vi "Post-Install Custom Action.vi"(10 "Variant":variant) -> (0 "error out":errorcluster)   [LabVIEW 2016]
uses:
  <vilib>/Utility/traverseref.llb/TRef TravTarget.ctl
  <vilib>/Utility/traverseref.llb/VI Scripting - Traverse.lvlib
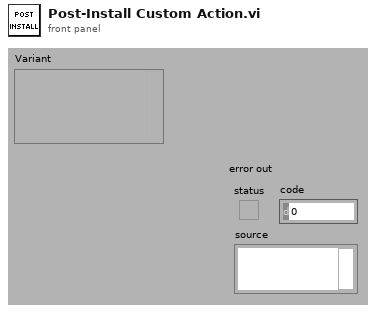
[diagram p1: front panel]
types:
  T1 = enum32{"Invalid", "Standard", "Closed", "Hidden", "Minimized", "Maximized"}
  T2 = typedef "TRef TravTarget.ctl" = enum16{"FP", "BD", "Other"}
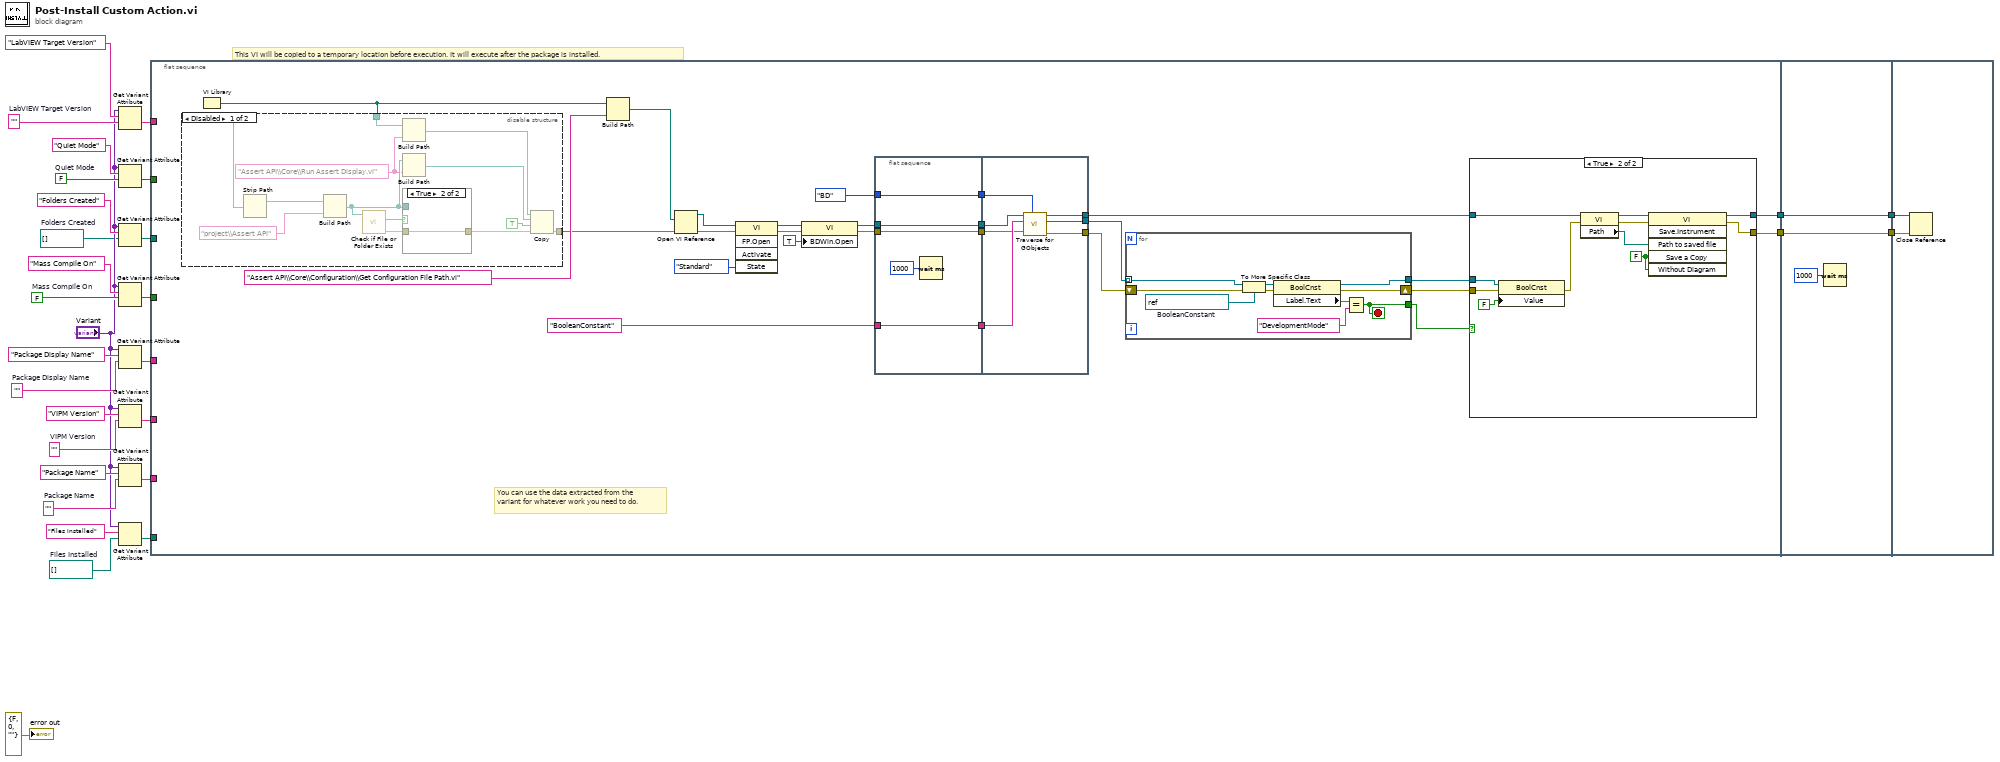
[diagram p0: block diagram]
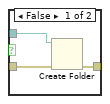
[diagram p2: hidden frame]
diagram:
  w5 = path[] []  # Folders Created
  w6 = path[] []  # Files Installed
  w12 = FALSE  # Mass Compile On
  w13 = ""  # Package Display Name
  w20 = FALSE  # Quiet Mode
  w23 = ""  # VIPM Version
  w25 = ""  # LabVIEW Target Version
  w27 = ""  # Package Name
  # "This VI will be copied to a temporary location before execution. It will execute after the package is installed."
  n1 = Get Variant Attribute(Variant="Variant", name="LabVIEW Target Version", default value (empty Variant)=w25) -> (value=w17:string)  [unwired: 1 in, 3 out]
  n2 = Get Variant Attribute(Variant="Variant", name="Quiet Mode", default value (empty Variant)=w20) -> (value=w15:bool)  [unwired: 1 in, 3 out]
  n3 = Get Variant Attribute(Variant="Variant", name="Folders Created", default value (empty Variant)=w5) -> (value=w10:path[])  [unwired: 1 in, 3 out]
  n4 = Get Variant Attribute(Variant="Variant", name="Mass Compile On", default value (empty Variant)=w12) -> (value=w14:bool)  [unwired: 1 in, 3 out]
  n5 = Get Variant Attribute(Variant="Variant", name="Package Display Name", default value (empty Variant)=w13) -> (value=w19:string)  [unwired: 1 in, 3 out]
  n6 = Get Variant Attribute(Variant="Variant", name="VIPM Version", default value (empty Variant)=w23) -> (value=w16:string)  [unwired: 1 in, 3 out]
  n7 = Get Variant Attribute(Variant="Variant", name="Package Name", default value (empty Variant)=w27) -> (value=w18:string)  [unwired: 1 in, 3 out]
  n8 = Get Variant Attribute(Variant="Variant", name="Files Installed", default value (empty Variant)=w6) -> (value=w9:path[])  [unwired: 1 in, 3 out]
  n9 = flat-sequence {
    tunnel: w19 -> [_]
    tunnel: w18 -> [_]
    tunnel: w17 -> [_]
    tunnel: w16 -> [_]
    tunnel: w15 -> [_]
    tunnel: w14 -> [_]
    tunnel: w9 -> [_]
    tunnel: w10 -> [_]
    tunnel: [w40] -> w3
    tunnel: [w39] -> w2
    tunnel: [w110] -> w4
    tunnel: w3 -> [w110]
    tunnel: w2 -> [w109]
    tunnel: [w109] -> w1
    tunnel: w4 -> [w112]
    tunnel: w1 -> [w111]
    frame #0 {
      # "Quiet Mode: This will indicate if VIPM is working in quiet mode.\nThis may happen if VIPM is running silently from the VIPM API.\nIf this is true then you should respect quiet mode and perform\nactions without any blocking dialog boxes or user prompts."
      # "You can use the data extracted from the variant for whatever work you need to do."
      n10 = VI Library() -> (path=w56:path)
      n11 = disable-structure shown="Disabled" {
        disable-tunnel: w56 -> [w70 _]
        disable-tunnel: [w69 _] -> w53
        frame Disabled {
          w75 = "Assert API\\Core\\Run Assert Display.vi" ("name or relative path")
          n12 = Strip Path(path=w70) -> (stripped path=w71:path)  [unwired: 1 out]
          n13 = Build Path(base path=w71, name or relative path="project\\Assert API") -> (appended path=w76:path)
          n14 = call <vilib>:"Check if File or Folder Exists.vi"("path"=w76) -> ("error out"=w77:errorcluster, "file or folder exists?"=w78:bool)  [unwired: 8 in, 1 out]
          n15 = Build Path(base path=w70, name or relative path=w75) -> (appended path=w80:path)
          n16 = Build Path(base path=w76, name or relative path=w75) -> (appended path=w74:path)
          n17 = case shown="True" w78 {
            tunnel: w76 -> [w83 _]
            tunnel: w77 -> [w82 w84]
            tunnel: [w81 w84] -> w72
            frame False {
              n18 = Create Folder(path (use dialog)=w83, error in=w82) -> (error out=w81:errorcluster)  [unwired: 1 in, 2 out]
            }
            frame True {
            }
          }
          n19 = Copy(8:w72, 9:TRUE ("overwrite (F)"), 10:w74, 11:w80) -> (0:w69:errorcluster)  [unwired: 1 in, 2 out]
        }
        frame Enabled {
        }
      }
      n20 = Build Path(base path=w56, name or relative path="Assert API\\Core\\Configuration\\Get Configuration File Path.vi") -> (appended path=w54:path)
      n21 = Open VI Reference(vi path=w54, error in (no error)=w53) -> (vi reference=w42:refnum<vi>, error out=w52:errorcluster)  [unwired: 4 in]
      n22 = invoke class="VI" method="FP.Open"(reference=w42, error in=w52, "State"=T1."Standard") -> (reference out=w37:refnum<vi>, error out=w43:errorcluster)  [unwired: 2 in, 3 out]
      n23 = property class="VI"(reference=w37, error in=w43, "BDWin.Open"=TRUE ("Block Diagram Window:Open")) -> (reference out=w36:refnum<vi>, error out=w38:errorcluster)
      n24 = flat-sequence {
        tunnel: w36 -> [w58]
        tunnel: w38 -> [w59]
        tunnel: "BooleanConstant" ("Class Name") -> [w60]
        tunnel: TRef_TravTarget."BD" ("Traverse Target") -> [w61]
        tunnel: [w61] -> w34
        tunnel: [w60] -> w33
        tunnel: [w59] -> w32
        tunnel: [w58] -> w31
        tunnel: [w66] -> w49
        tunnel: [w65] -> w45
        tunnel: [w64] -> w44
        tunnel: w34 -> [w68]
        tunnel: w33 -> [w67]
        tunnel: w32 -> [w63]
        tunnel: w31 -> [w62]
        frame #0 {
          n25 = Wait (ms)(milliseconds to wait=u32 1000) -> ()  [unwired: 1 out]
        }
        frame #1 {
          n26 = call <vilib>:"Traverse for GObjects.vi"("Traverse Target"=w68, "error in (no error)"=w63, "Class Name"=w67, "VI Refnum"=w62) -> ("error out"=w65:errorcluster, "References"=w66:refnum<vi>[], "dup VI Refnum"=w64:refnum<vi>)  [unwired: 4 in, 1 out]
        }
      }
      n27 = for {
        tunnel: w49 -> [w107] mode=indexing
        tunnel: [w102] -> w47
        tunnel: [w101] -> w48
        shift-right: [w100] -> w46
        shift-left: w45 -> [w99]
        stop <- w101 stop-if-true
        w105 = refnum<vi> refnum  # BooleanConstant
        n28 = To More Specific Class(target class=w105, reference=w107, error in=w99) -> (specific class reference=w106:refnum<vi>, error out=w98:errorcluster)
        n29 = property class="BoolCnst"(reference=w106, error in=w98) -> (reference out=w102:refnum<vi>, error out=w100:errorcluster, "Label.Text"=w104:string)
        n30 = Equal?(x=w104, y="DevelopmentMode") -> (x = y?=w101:bool)
      }
      n31 = case shown="True" w48 {
        tunnel: w47 -> [_ w97]
        tunnel: w46 -> [w85 w95]
        tunnel: w44 -> [w86 w94]
        tunnel: [w85 w88] -> w39
        tunnel: [w86 w87] -> w40
        frame False {
        }
        frame True {
          w89 = FALSE ("Save a Copy")
          n32 = property class="BoolCnst"(reference=w97, error in=w95, "Value"=FALSE) -> (error out=w93:errorcluster)  [unwired: 1 out]
          n33 = property class="VI"(reference=w94, error in=w93) -> (reference out=w91:refnum<vi>, error out=w92:errorcluster, "Path"=w90:path)
          n34 = invoke class="VI" method="Save.Instrument"(reference=w91, error in=w92, "Path to saved file"=w90, "Save a Copy"=w89, "Without Diagram"=w89) -> (reference out=w87:refnum<vi>, error out=w88:errorcluster)  [unwired: 1 in, 4 out]
        }
      }
    }
    frame #1 {
      n35 = Wait (ms)(milliseconds to wait=u32 1000) -> ()  [unwired: 1 out]
    }
    frame #2 {
      n36 = Close Reference(reference=w112, error in (no error)=w111) -> ()  [unwired: 1 out]
    }
  }
  "error out" <- errorcluster {"status"=FALSE, "code"=0, "source"=""} ("error out")
